vi "sub_ch-start-finish.vi"(7 "cmd":enum16{"Start", "Finish"}(ring), 8 "error in":errorcluster, 10 "repeat":i32, 11 "Ch":i32) -> (0 "error out":errorcluster, 2 "dt(ms)":u32, 3 "HWseq-array":T1[](array[typedef]))   [LabVIEW 2019]
uses:
  Capacitor/rc-seq_enum.ctl
  SubVIs/cmd_timer.ctl
  _ctrl/rw.ctl
  _ctrl/fgv_DL950.ctl
  SubVIs/common/hw-control.ctl
  SubVIs/common/_ctrl/system-status.ctl
  Capacitor/measure_rc.ctl
  result.ctl
  cmd_timecheck.ctl
  _ctrl/init-r-stop.ctl
  Capacitor/breakdown.ctl
  log save type.ctl
  _ctrl/create-rw-close.ctl
  SubVIs/common/Glob_Ref.vi
  Global 1.vi
  _ctrl/init-r-w.ctl
  SubVIs/common/cmd_tablecnt.ctl
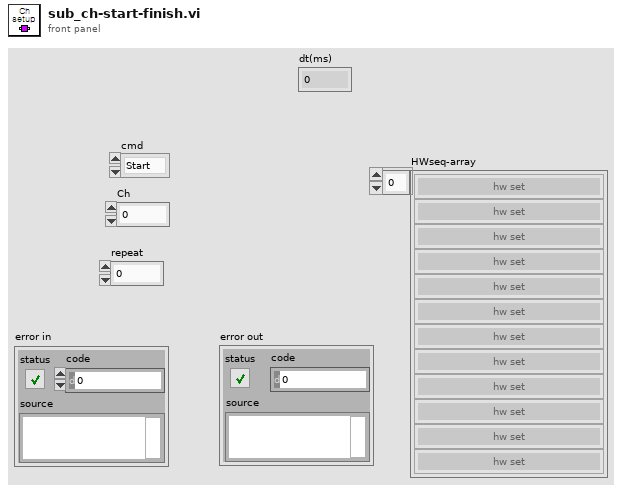
[diagram p1: front panel]
types:
  T1 = typedef "rc-seq_enum.ctl" = enum16{"hw set", "Pwr-in on", "ch-relay on", "Pwr-out on", "AO on", "AO 0v", "Pwr-in off", "Relay-all off", "Pwr-out off", "Discharge", "950 read", "Run", "Stop"}
  T2 = typedef "cmd_timer.ctl" = enum16{"init", "init_update", "run", "default", "update"}
  T3 = typedef "fgv_DL950.ctl" = enum16{"init", "config", "Set-NCh", "setapply", "trigger", "history_clear", "read", "time-div", "wave-aquis", "start", "query", "abort", "set_items", "reset_items", "read_items", "percent_rise", "trigger_single", "stop", "offset cancel", "close"}
  T4 = typedef "rw.ctl" = enum16{"read", "write"}
  T5 = typedef "hw-control.ctl" = enum16{"DL950 ready", "DL950 clear", "DL950 trigger", "DL950 read", "DL950 read seq", "DL950 Tsingle query", "AO 12v", "AO wave", "AO 0v", "relay all-off", "Discharge check", "Discharge", "Relay1", "Relay2", "Relay3", "Relay4", "Relay5", "Relay6", "BP4610 onoff", "BP4610 set", "DSP1500 set", "DSP1500 onoff"}
  T6 = typedef "system-status.ctl" = enum16{"Initial", "Update", "Clear", "Read"}
  T7 = typedef "measure_rc.ctl" = cluster{"입력카운트":dbl, "출력카운트":dbl, "Rising Time 63%":dbl, "Rising Time 98%":dbl, "Failing Time 37%":dbl, "입력전류 RMS":dbl, "출력전류 RMS":dbl, "출력전압 + 평균 63%":dbl, "출력전압 - 평균 63%":dbl, "출력전류 평균 63%":dbl, "접촉저항":dbl, "온도":dbl, "충전전압 63초":dbl, "충전전압 98초":dbl, "충전전류 37초":dbl, "방전전압":dbl, "전압강하":dbl, "부하전압(고장)":dbl}
  T8 = typedef "result.ctl" = enum16{"Init", "OK", "NG", "Shutdown", "Testing", "Completion", "Device Error", "Start", "작동", "미작동", "작동 대기", "작동 1"}
  T9 = typedef "cmd_timecheck.ctl" = enum16{"Group start", "Group end", "Grout dt", "Ch start", "Ch end", "Ch dt", "init", "NF start", "NF stop", "idrc start", "idrc stop", "scope start", "scope stop", "ao start", "ao stop", "relay start", "relay stop", "NF read start", "NF read stop", "NF set start", "NF set stop", "idrc level start", "idrc level stop", "scope trig start", "scope trig stop", "relay dischar star", "relay dischar stop", "data process start", "data process stop", "ch-relay on start", "ch-relay on stop", "hw set start", "hw set stop", "pwr-in on start", "pwr-in on stop", "pwr-out on start", "pwr-out on stop", "ao on start", "ao on stop", "ao 0v start", "ao 0v stop", "pwr-in off start", "pwr-in off stop", "relay-all off start", "relay-all off stop", "pwr-out off start", "pwr-out off stop", "discharge start", "discharge stop", "950 read start", "950 read stop"}
  T10 = typedef "init-r-stop.ctl" = enum16{"ini", "read", "stop"}
  T11 = typedef "init-r-w.ctl" = enum16{"init", "read", "write"}
  T12 = typedef "breakdown.ctl" = enum16{"DL950 items", "input pwr", "output pwr"}
  T13 = typedef "log save type.ctl" = enum16{"header", "data"}
  T14 = typedef "create-rw-close.ctl" = enum16{"create", "write", "read", "delete", "close"}
  T15 = typedef "cmd_tablecnt.ctl" = enum16{"Create", "Inital", "Write", "Default"}
  T16 = typedef "Testing-info.ctl" = cluster{"전체채널수":u8, "현재채널번호":u8, "Irms":dbl, "입력전압":dbl, "입력전류":dbl, "출력전압":dbl, "출력전류":dbl, "온도":dbl, "제어단 단선":bool, "제어단 단락":bool, "제어단 특성변화":bool, "출력단 단선":bool, "출력단 단락":bool, "출력단 특성변화":bool, "출력단 전압":bool, "카운트 일치":bool, "Irms 판정":bool, "온도":bool, "테스트 회수":u32, "TestType":T17, "현재회수":u32, "Ch selection":cluster{"1ch":bool, "2ch":bool, "3ch":bool, "4ch":bool, "5ch":bool, "6ch":bool}, "반복":u32, "Path":path, "파일생성주기":u32, "start time":dbl, "stop time":dbl, "현재반복회수":u32, "NG":cluster{"입출력 카운트":bool, "출력전류RMS":bool}}
  T17 = typedef "sequence_single.ctl" = enum16{"Register", "RC", "B1", "B2", "B3", "Oper_LV", "Oper_HV", "ContR_LV"}
  T18 = typedef "error_rc.ctl" = cluster{"제어단 단선":bool, "제어단 단락":bool, "제어단 특성변화":bool, "출력단 단선":bool, "출력단 단락":bool, "출력단 특성변화":bool, "출력전압":bool, "카운트 일치":bool, "전압 98%":bool, "전압 63%":bool, "전류 37%":bool, "방전전압":bool, "온도":bool}
  T19 = typedef "result-path.ctl" = cluster{"Path-arr":path[]}
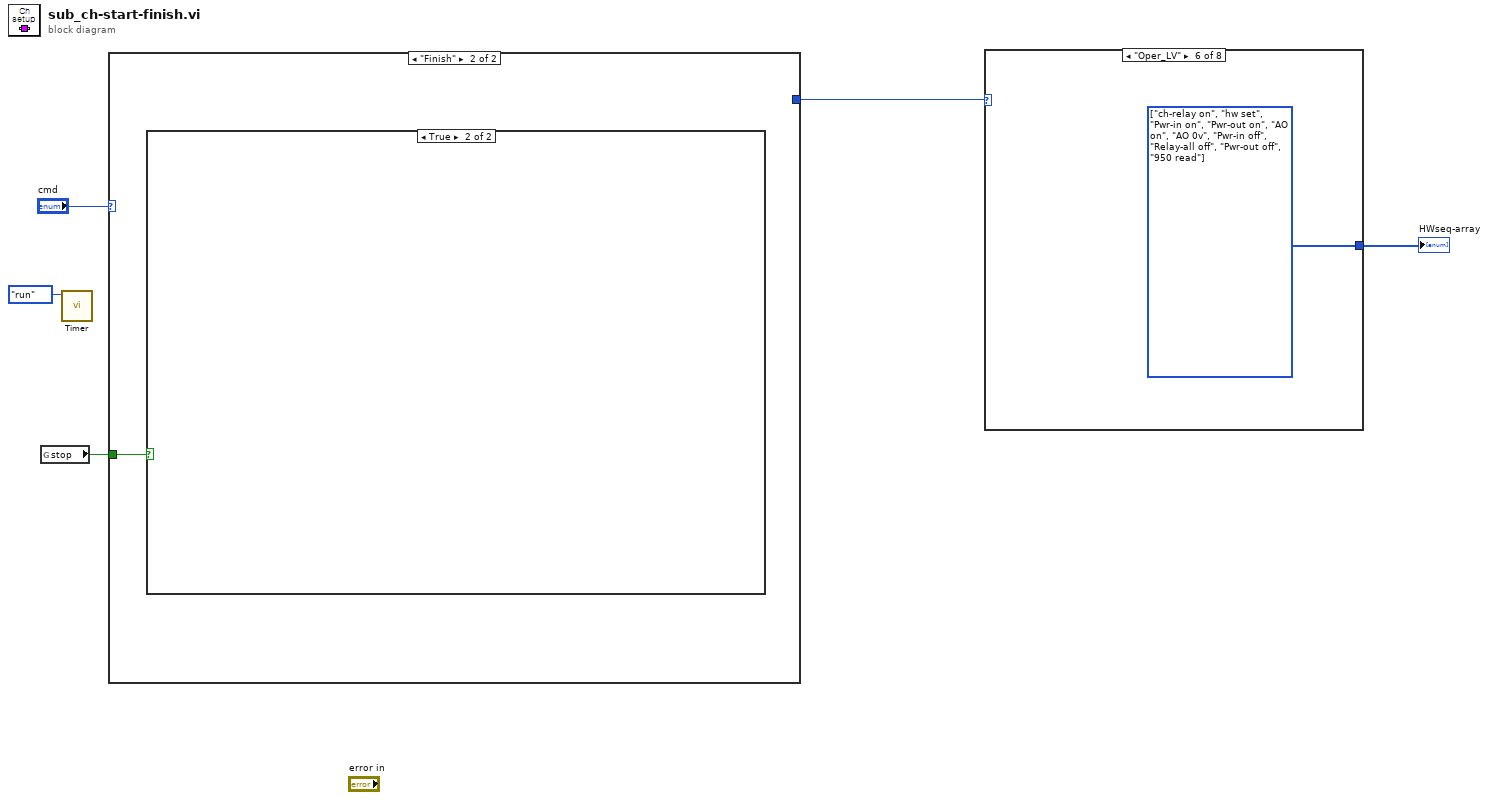
[diagram p0: block diagram]
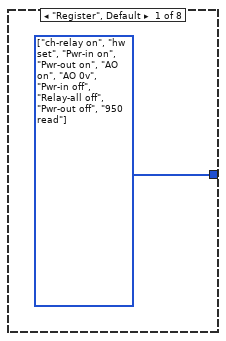
[diagram p2: hidden frame]
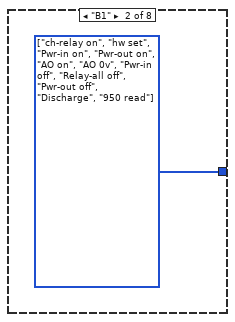
[diagram p3: hidden frame]
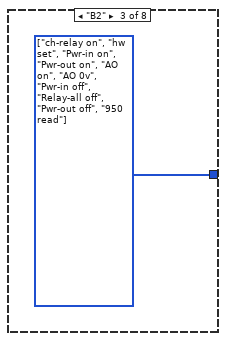
[diagram p4: hidden frame]
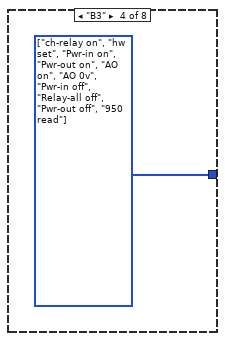
[diagram p5: hidden frame]
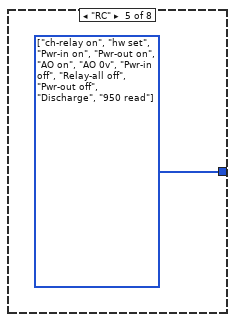
[diagram p6: hidden frame]
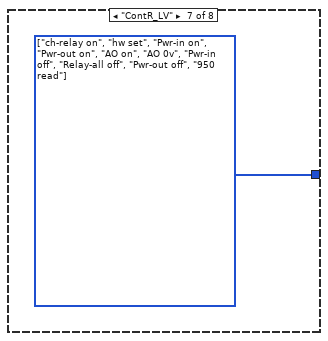
[diagram p7: hidden frame]
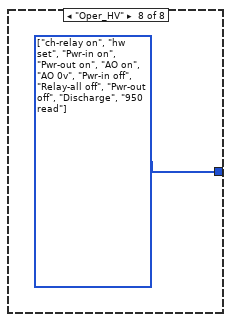
[diagram p8: hidden frame]
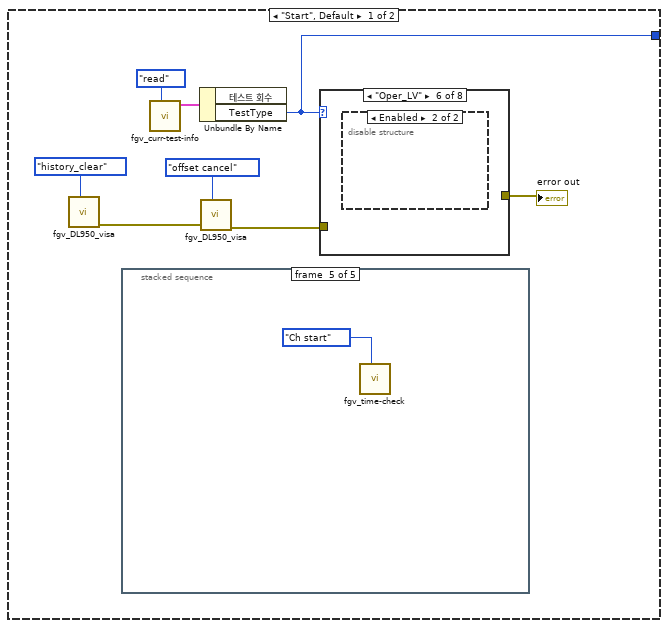
[diagram p9: hidden frame]
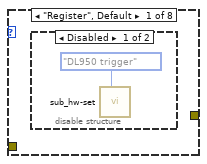
[diagram p10: hidden frame]
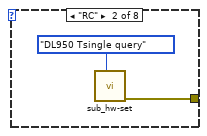
[diagram p12: hidden frame]
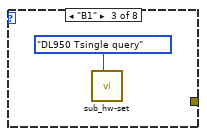
[diagram p13: hidden frame]
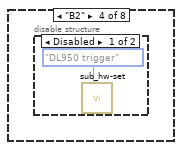
[diagram p14: hidden frame]
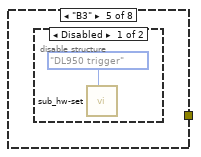
[diagram p16: hidden frame]
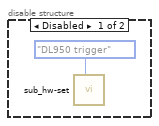
[diagram p18: hidden frame]
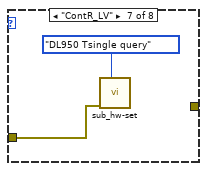
[diagram p19: hidden frame]
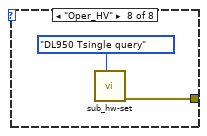
[diagram p20: hidden frame]
diagram:
  n1 = global read "Glob_Ref.vi" "stop"() -> (w2:bool)
  n2 = call "Timer.vi"("cmd"=cmd_timer."run") -> ()  [unwired: 8 in, 3 out]
  n3 = case shown="\"Finish\"" "cmd" {
    tunnel: [w10 _] -> w4
    tunnel: w2 -> [_ w48]
    frame "Start", Default {
      n4 = call "fgv_DL950_visa.vi"("cmd"=fgv_DL950."history_clear") -> ("error out"=w7:errorcluster)  [unwired: 8 in, 2 out]
      n5 = stacked-sequence {
        frame #0 {
          n6 = Increment(x="Ch") -> (x+1=w28:i32)
          n7 = Number To Decimal String(number=w28) -> (decimal integer string=w25:string)  [unwired: 1 in]
          n8 = call "fgv_curr-test-info.vi"("cmd"=rw."read") -> ("현재테스트 정보 2"=w31:T16)  [unwired: 10 in]
          n9 = Bundle By Name(cluster=w31, "현재채널번호"="Ch") -> (w32:T16)
          n10 = call "fgv_curr-test-info.vi"("cmd"=rw."write", "현재테스트 정보"=w32) -> ()  [unwired: 9 in, 1 out]
          n11 = call "sub_log_basic.vi"("desc"=w25, "Title"="Test Channel") -> ()  [unwired: 9 in, 1 out]
          n12 = call "fgv_status-display.vi"("Mode"=system-status."Update", "detail"=w25, "title"="\n>>Curr channel ----") -> ()  [unwired: 8 in, 1 out]
        }
        frame #1 {
          n13 = Increment(x="repeat") -> (x+1=w37:i32)
          n14 = call "fgv_curr-test-info.vi"("cmd"=rw."read") -> ("현재테스트 정보 2"=w40:T16)  [unwired: 10 in]
          n15 = Bundle By Name(cluster=w40, "현재반복회수"="repeat") -> (w41:T16)
          n16 = Number To Decimal String(number=w37) -> (decimal integer string=w35:string)  [unwired: 1 in]
          n17 = call "fgv_curr-test-info.vi"("cmd"=rw."write", "현재테스트 정보"=w41) -> ()  [unwired: 9 in, 1 out]
          n18 = call "fgv_status-display.vi"("Mode"=system-status."Update", "detail"=w35, "title"="\n//repeat no") -> ()  [unwired: 8 in, 1 out]
        }
        frame #2 {
          n19 = call "fgv_measure_rc.vi"("cmd"=rw."write", "measure_rc"=T7 {"입력카운트"=0.0, "출력카운트"=0.0, "Rising Time 63%"=0.0, "Rising Time 98%"=0.0, "Failing Time 37%"=0.0, "입력전류 RMS"=0.0, "출력전류 RMS"=0.0, "출력전압 + 평균 63%"=0.0, "출력전압 - 평균 63%"=0.0, "출력전류 평균 63%"=0.0, "접촉저항"=0.0, "온도"=0.0, "충전전압 63초"=0.0, "충전전압 98초"=0.0, "충전전류 37초"=0.0, "방전전압"=0.0, "전압강하"=0.0, "부하전압(고장)"=0.0}) -> ()  [unwired: 9 in, 1 out]
        }
        frame #3 {
          # "Result UI"
          n20 = call "UI_result.vi"("result"=result."Testing") -> ()  [unwired: 10 in, 1 out]
        }
        frame #4 {
          n21 = call "fgv_time-check.vi"("cmd"=cmd_timecheck."Ch start") -> ()  [unwired: 9 in, 2 out]
        }
      }
      n22 = call "fgv_curr-test-info.vi"("cmd"=rw."read") -> ("현재테스트 정보 2"=w13:T16)  [unwired: 10 in]
      n23 = Unbundle By Name(w13) -> ("TestType"=w10:T17)  [unwired: 1 out]
      n24 = call "fgv_DL950_visa.vi"("cmd"=fgv_DL950."offset cancel", "error in"=w7) -> ("error out"=w6:errorcluster)  [unwired: 7 in, 2 out]
      n25 = case shown="\"Oper_LV\"" w10 {
        tunnel: [_ w15 _ _ _ _ _ w23] -> w11
        tunnel: w6 -> [_ _ _ _ _ _ w21 _]
        frame "Register", Default {
          n26 = disable-structure shown="Disabled" {
            frame Disabled {
              n27 = call "sub_hw-set.vi"("cmd"=hw-control."DL950 trigger") -> ()  [unwired: 10 in, 1 out]
            }
            frame Enabled {
            }
          }
        }
        frame "RC" {
          n28 = call "sub_hw-set.vi"("cmd"=hw-control."DL950 Tsingle query") -> ("error out"=w15:errorcluster)  [unwired: 10 in]
        }
        frame "B1" {
          n29 = call "sub_hw-set.vi"("cmd"=hw-control."DL950 Tsingle query") -> ()  [unwired: 10 in, 1 out]
        }
        frame "B2" {
          n30 = disable-structure shown="Disabled" {
            frame Disabled {
              n31 = call "sub_hw-set.vi"("cmd"=hw-control."DL950 trigger") -> ()  [unwired: 10 in, 1 out]
            }
            frame Enabled {
            }
          }
        }
        frame "B3" {
          n32 = disable-structure shown="Disabled" {
            frame Disabled {
              n33 = call "sub_hw-set.vi"("cmd"=hw-control."DL950 trigger") -> ()  [unwired: 10 in, 1 out]
            }
            frame Enabled {
            }
          }
        }
        frame "Oper_LV" {
          n34 = disable-structure shown="Enabled" {
            frame Disabled {
              n35 = call "sub_hw-set.vi"("cmd"=hw-control."DL950 trigger") -> ()  [unwired: 10 in, 1 out]
            }
            frame Enabled {
            }
          }
        }
        frame "ContR_LV" {
          n36 = call "sub_hw-set.vi"("cmd"=hw-control."DL950 Tsingle query", "error in"=w21) -> ()  [unwired: 9 in, 1 out]
        }
        frame "Oper_HV" {
          n37 = call "sub_hw-set.vi"("cmd"=hw-control."DL950 Tsingle query") -> ("error out"=w23:errorcluster)  [unwired: 10 in]
        }
      }
      "error out" <- w11
    }
    frame "Finish" {
      n38 = case shown="True" w48 {
        frame False {
          n39 = stacked-sequence {
            seq-local: [w50 _ _ _ _ _ _ _] -> [_ _ _ _ _ w84 _ _]
            frame #0 {
              n40 = disable-structure shown="Disabled" {
                frame Disabled {
                  n41 = call "fgv_DL950_visa.vi"("cmd"=fgv_DL950."offset cancel") -> ()  [unwired: 8 in, 3 out]
                }
                frame Enabled {
                }
              }
              n42 = call "fgv_time-check.vi"("cmd"=cmd_timecheck."data process start") -> ()  [unwired: 9 in, 2 out]
              n43 = Tick Count (ms)() -> (millisecond timer value=w50:u32)
            }
            frame #1 {
              n44 = call "fgv_stop_local.vi"("cmd"=init-r-stop."read") -> ()  [unwired: 9 in, 2 out]
              n45 = case shown="True" TRUE {
                frame False {
                  n46 = call "fgv_error_rc.vi"("cmd"=init-r-w."read") -> ("Error 2"=w60:T18)  [unwired: 10 in]
                  n47 = Cluster To Array(cluster=w60) -> (array=w59:bool[])
                  n48 = Or Array Elements(Boolean array=w59) -> (logical OR=w57:bool)
                  n49 = Select(t=result."NG" ("result"), s=w57, f=result."OK" ("result")) -> (s? t:f=w56:T8)
                  n50 = call "UI_result.vi"("result"=w56) -> ()  [unwired: 10 in, 1 out]
                }
                frame True {
                  # "shutdown"
                }
              }
            }
            frame #2 {
              # "update result"
              n51 = call "sub_result-update.vi"() -> ()  [unwired: 12 in]
            }
            frame #3 {
              # "판정"
              n52 = call "sub_breakdown-check.vi"("breakdown type"=breakdown."DL950 items") -> ()  [unwired: 10 in, 1 out]
            }
            frame #4 {
              # "결과저장"
              n53 = case shown="False" FALSE {
                frame False {
                  n54 = call "sub_log-header-write.vi"("cmd"=log_save_type."data") -> ()  [unwired: 10 in, 1 out]
                }
                frame True {
                  n55 = call "TableCnt.vi"("cnt"=cmd_tablecnt."Default") -> ("Item Names"=w68:string[][])  [unwired: 9 in, 1 out]
                  n56 = Array To Spreadsheet String(array=w68, 3:"" ("format string")) -> (spreadsheet string=w65:string)  [unwired: 1 in]
                  n57 = disable-structure shown="Disabled" {
                    disable-tunnel: w65 -> [w70 _]
                    frame Disabled {
                      n58 = call "fgv_save-info.vi"("cmd"=rw."read") -> ("save info 2"=w80:T19)  [unwired: 10 in]
                      n59 = call "fgv_curr-test-info.vi"("cmd"=rw."read") -> ("현재테스트 정보 2"=w77:T16)  [unwired: 10 in]
                      n60 = Unbundle By Name(w77) -> ("현재채널번호"=w76:u8)
                      n61 = Unbundle By Name(w80) -> ("Path-arr"=w79:path[])
                      n62 = Index Array(array=w79, index=w76) -> (element=w73:path)
                      n63 = Open/Create/Replace File(file path (use dialog)=w73) -> (refnum out=w75:refnum<file>, error out=w72:errorcluster)  [unwired: 5 in, 1 out]
                      n64 = Write to Text File(file (use dialog)=w75, text=w70, error in=w72) -> (refnum out=w74:refnum<file>, error out=w71:errorcluster)  [unwired: 1 in, 1 out]
                      n65 = Close File(refnum=w74, error in=w71) -> ()  [unwired: 2 out]
                    }
                    frame Enabled {
                    }
                  }
                  n66 = To Variant(anything=w65) -> (Variant=w64:variant)
                  n67 = call "fgv-data.vi"("cmd"=create-rw-close."write", "element"=w64) -> ()  [unwired: 8 in, 2 out]
                }
              }
            }
            frame #5 {
              n68 = Tick Count (ms)() -> (millisecond timer value=w85:u32)
              n69 = Subtract(x=w85, y=w84) -> (x-y=w83:u32)
              "dt(ms)" <- w83
              n70 = global write "Global 1.vi" "dt(ms)_finish"(w83) -> ()
              n71 = call "fgv_DL950_q.vi"("cmd"=create-rw-close."delete") -> ()  [unwired: 9 in, 2 out]
            }
            frame #6 {
            }
            frame #7 {
              w92 = "-------" ("desc")
              w91 = ">>Ch finish" ("title")
              n72 = call "fgv_status-display.vi"("Mode"=system-status."Update", "detail"=w92, "title"=w91) -> ("error out"=w86:errorcluster)  [unwired: 8 in]
              n73 = call "sub_log_basic.vi"("desc"=w92, "Title"=w91) -> ()  [unwired: 9 in, 1 out]
              n74 = call "fgv_time-check.vi"("cmd"=cmd_timecheck."data process stop", "error in (no error)"=w86) -> ("error out"=w89:errorcluster)  [unwired: 8 in, 1 out]
              n75 = call "fgv_time-check.vi"("cmd"=cmd_timecheck."Ch end", "error in (no error)"=w89) -> ()  [unwired: 8 in, 2 out]
            }
          }
        }
        frame True {
        }
      }
    }
  }
  n76 = case shown="\"Oper_LV\"" w4 {
    tunnel: [w93 w94 w95 w96 w97 w98 w99 w100] -> w3
    frame "Register", Default {
      w93 = T1[] [enum."ch-relay on", enum."hw set", enum."Pwr-in on", enum."Pwr-out on", enum."AO on", enum."AO 0v", enum."Pwr-in off", enum."Relay-all off", enum."Pwr-out off", enum."950 read"] items=["hw set", "Pwr-in on", "ch-relay on", "Pwr-out on", "AO on", "AO 0v", "Pwr-in off", "Relay-all off", "Pwr-out off", "Discharge", "950 read", "Run", "Stop"]
    }
    frame "B1" {
      w94 = T1[] [enum."ch-relay on", enum."hw set", enum."Pwr-in on", enum."Pwr-out on", enum."AO on", enum."AO 0v", enum."Pwr-in off", enum."Relay-all off", enum."Pwr-out off", enum."Discharge", enum."950 read"] items=["hw set", "Pwr-in on", "ch-relay on", "Pwr-out on", "AO on", "AO 0v", "Pwr-in off", "Relay-all off", "Pwr-out off", "Discharge", "950 read", "Run", "Stop"]
    }
    frame "B2" {
      w95 = T1[] [enum."ch-relay on", enum."hw set", enum."Pwr-in on", enum."Pwr-out on", enum."AO on", enum."AO 0v", enum."Pwr-in off", enum."Relay-all off", enum."Pwr-out off", enum."950 read"] items=["hw set", "Pwr-in on", "ch-relay on", "Pwr-out on", "AO on", "AO 0v", "Pwr-in off", "Relay-all off", "Pwr-out off", "Discharge", "950 read", "Run", "Stop"]
    }
    frame "B3" {
      w96 = T1[] [enum."ch-relay on", enum."hw set", enum."Pwr-in on", enum."Pwr-out on", enum."AO on", enum."AO 0v", enum."Pwr-in off", enum."Relay-all off", enum."Pwr-out off", enum."950 read"] items=["hw set", "Pwr-in on", "ch-relay on", "Pwr-out on", "AO on", "AO 0v", "Pwr-in off", "Relay-all off", "Pwr-out off", "Discharge", "950 read", "Run", "Stop"]
    }
    frame "RC" {
      w97 = T1[] [enum."ch-relay on", enum."hw set", enum."Pwr-in on", enum."Pwr-out on", enum."AO on", enum."AO 0v", enum."Pwr-in off", enum."Relay-all off", enum."Pwr-out off", enum."Discharge", enum."950 read"] items=["hw set", "Pwr-in on", "ch-relay on", "Pwr-out on", "AO on", "AO 0v", "Pwr-in off", "Relay-all off", "Pwr-out off", "Discharge", "950 read", "Run", "Stop"]
    }
    frame "Oper_LV" {
      w98 = T1[] [enum."ch-relay on", enum."hw set", enum."Pwr-in on", enum."Pwr-out on", enum."AO on", enum."AO 0v", enum."Pwr-in off", enum."Relay-all off", enum."Pwr-out off", enum."950 read"] items=["hw set", "Pwr-in on", "ch-relay on", "Pwr-out on", "AO on", "AO 0v", "Pwr-in off", "Relay-all off", "Pwr-out off", "Discharge", "950 read", "Run", "Stop"]
    }
    frame "ContR_LV" {
      w99 = T1[] [enum."ch-relay on", enum."hw set", enum."Pwr-in on", enum."Pwr-out on", enum."AO on", enum."AO 0v", enum."Pwr-in off", enum."Relay-all off", enum."Pwr-out off", enum."950 read"] items=["hw set", "Pwr-in on", "ch-relay on", "Pwr-out on", "AO on", "AO 0v", "Pwr-in off", "Relay-all off", "Pwr-out off", "Discharge", "950 read", "Run", "Stop"]
    }
    frame "Oper_HV" {
      w100 = T1[] [enum."ch-relay on", enum."hw set", enum."Pwr-in on", enum."Pwr-out on", enum."AO on", enum."AO 0v", enum."Pwr-in off", enum."Relay-all off", enum."Pwr-out off", enum."Discharge", enum."950 read"] items=["hw set", "Pwr-in on", "ch-relay on", "Pwr-out on", "AO on", "AO 0v", "Pwr-in off", "Relay-all off", "Pwr-out off", "Discharge", "950 read", "Run", "Stop"]
    }
  }
  "HWseq-array" <- w3
